vi "PWMToAngle.vi"(10 "offset":dbl, 11 "input":dbl) -> (3 "angle (radians)":dbl)   [LabVIEW 2013]
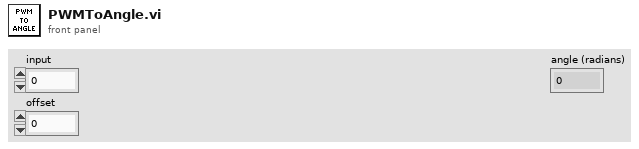
[diagram p1: front panel]
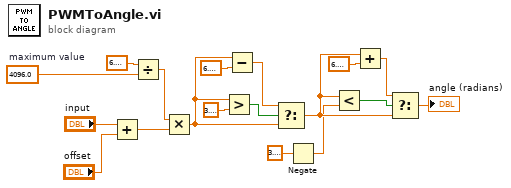
[diagram p0: block diagram]
diagram:
  w17 = 4096.0  # maximum value
  n1 = Add(x="input", y="offset") -> (x+y=w2:dbl)
  n2 = Divide(x=6.283185307179586, y=w17) -> (x/y=w16:dbl)
  n3 = Multiply(x=w16, y=w2) -> (x*y=w1:dbl)
  n4 = Greater?(x=w1, y=3.141592653589793) -> (0:w15:bool)
  n5 = Subtract(x=w1, y=6.283185307179586) -> (x-y=w12:dbl)
  n6 = Select(t=w12, s=w15, f=w1) -> (s? t:f=w8:dbl)
  n7 = Negate(x=3.141592653589793) -> (-x=w5:dbl)
  n8 = Less?(x=w8, y=w5) -> (x < y?=w6:bool)
  n9 = Add(x=w8, y=6.283185307179586) -> (x+y=w11:dbl)
  n10 = Select(t=w11, s=w6, f=w8) -> (s? t:f=→"angle (radians)":dbl)
